vi "ChangeServoPosition.vi"(5 "Position Log Ref":refnum<k34>, 6 "Close communication":bool, 7 "Communication Log Ref":refnum<file>, 8 "error in (no error)":errorcluster, 9 "Value":i16, 10 "Label.Text":string, 11 "VISA Refnum in":refnum<visa-resource-name>) -> (0 "error out":errorcluster, 3 "VISA resource name out":refnum<visa-resource-name>)   [LabVIEW 2018]
doc: "Send command to change servo position and write communication message to log file."
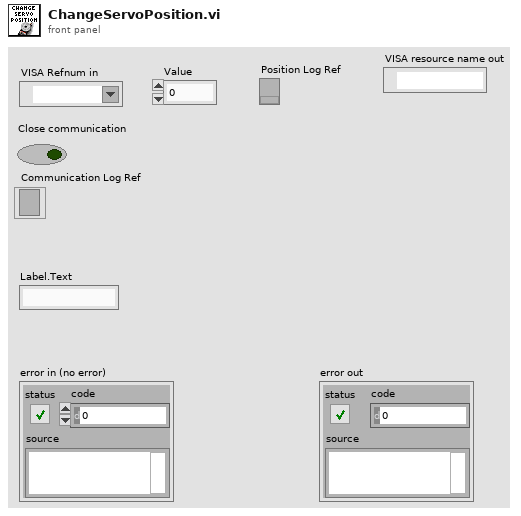
[diagram p1: front panel]
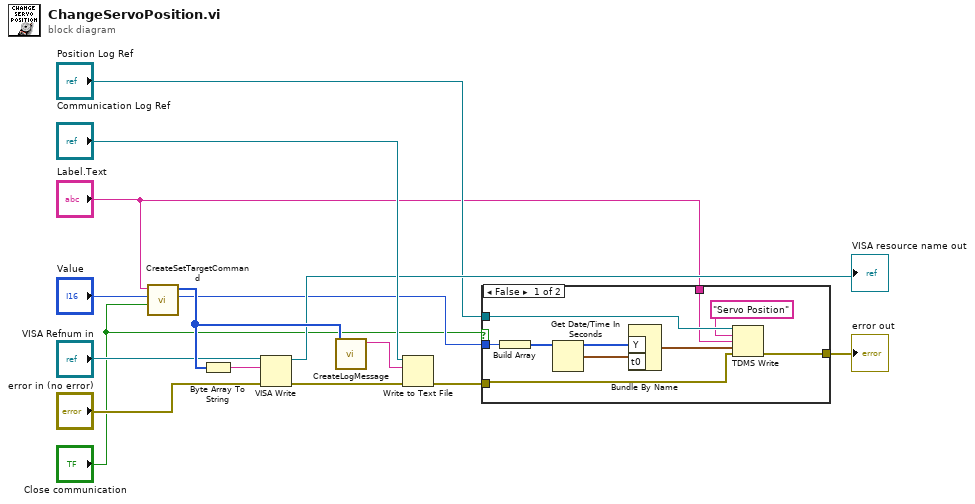
[diagram p0: block diagram]
diagram:
  n1 = call "CreateSetTargetCommand.vi"("Close communication"="Close communication", "Target value"="Value", "Sevo name"="Label.Text") -> ("Command"=w13:u32[])  [unwired: 8 in]
  n2 = Byte Array To String(unsigned byte array=w13) -> (string=w12:string)
  n3 = VISA Write(VISA resource name="VISA Refnum in", write buffer=w12, error in (no error)="error in (no error)") -> (VISA resource name out=→"VISA resource name out":refnum<visa-resource-name>, error out=w14:errorcluster)  [unwired: 1 out]
  n4 = call "CreateLogMessage.vi"("Command byte array"=w13) -> ("Log Message"=w11:string)  [unwired: 10 in]
  n5 = Write to Text File(file (use dialog)="Communication Log Ref", text=w11, error in=w14) -> (error out=w3:errorcluster)  [unwired: 1 in, 2 out]
  n6 = case shown="False" "Close communication" {
    tunnel: "Position Log Ref" -> [w23 _]
    tunnel: "Label.Text" -> [w20 _]
    tunnel: "Value" -> [w18 _]
    tunnel: w3 -> [w16 w24]
    tunnel: [w15 w24] -> w2
    frame False {
      n7 = Build Array(w18) -> (w17:i16[])
      n8 = Get Date/Time In Seconds() -> (seconds since 1Jan1904=w19:timestamp)
      n9 = Bundle By Name("Y"=w17, "t0"=w19) -> (w21:waveform(i16))  [unwired: 1 in]
      n10 = TDMS Write(0:w23, 5:"Servo Position" ("group name in (Untitled)"), 7:w20, 9:w21, 11:w16) -> (15:w15:errorcluster)  [unwired: 1 in, 3 out]
    }
    frame True {
    }
  }
  "error out" <- w2
